vi "Init.vi"(8 "error in (no error)":errorcluster, 10 "ID":string, 11 "Spring Motor in":refnum<class "Spring Motor.lvclass">) -> (0 "error out":errorcluster, 3 "Spring Motor out":refnum<class "Spring Motor.lvclass">)   [LabVIEW 2021, in "Spring Motor.lvclass"]
uses:
  Spring Motor.lvclass
  Spring Motor.lvclass/Spring Motor.ctl
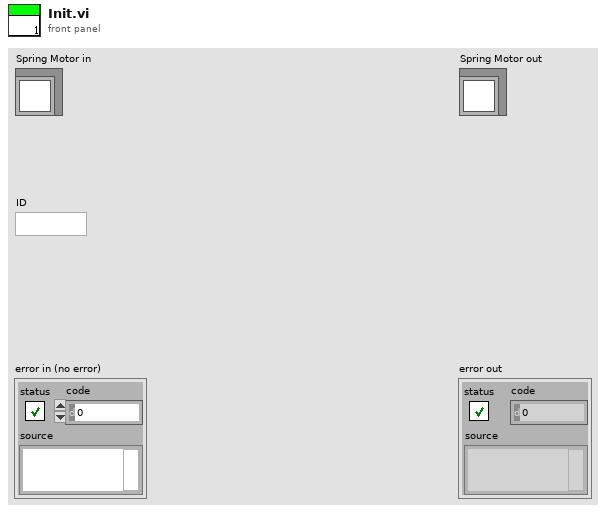
[diagram p1: front panel]
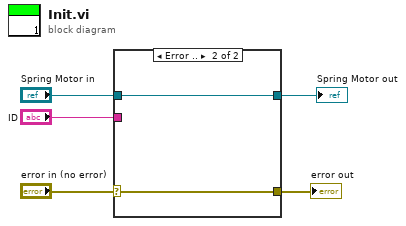
[diagram p0: block diagram]
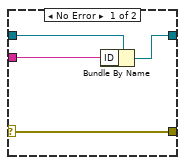
[diagram p2: hidden frame]
diagram:
  n1 = case shown="Error .." "error in (no error)" {
    selector: "error in (no error)" -> [w7 w11]
    tunnel: [w9 w10] -> w5
    tunnel: "Spring Motor in" -> [w8 w10]
    tunnel: [w7 w11] -> w2
    tunnel: "ID" -> [w6 _]
    frame No Error {
      n2 = Bundle By Name(cluster=w8, "ID"=w6) -> (w9:refnum<class "Spring Motor.lvclass">)
    }
    frame Error {
    }
  }
  "error out" <- w2
  "Spring Motor out" <- w5
